vi "GetObjectivePosition.vi"(8 "error in (no error)":errorcluster) -> (0 "error out":errorcluster, 1 "output cluster":cluster{"X":dbl, "Y":dbl, "Z":dbl}, 2 "Valid":bool, 3 "CurrentPosition":cluster{"X":dbl, "Y":dbl, "Z":dbl, "Depth":dbl})   [LabVIEW 2014]
panel:
  out "Stale":bool
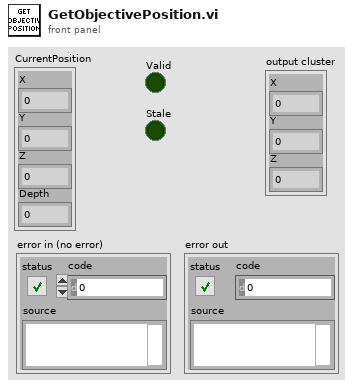
[diagram p1: front panel]
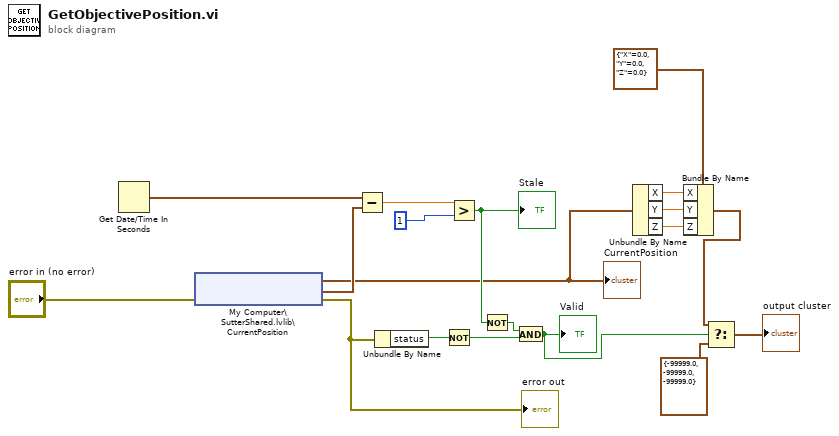
[diagram p0: block diagram]
diagram:
  n1 = Get Date/Time In Seconds() -> (seconds since 1Jan1904=w19:timestamp)
  n2 = shared-variable "My Computer\\SutterShared.lvlib\\CurrentPosition"(error in="error in (no error)") -> (w9:cluster{"X":dbl, "Y":dbl, "Z":dbl, "Depth":dbl}, error out=w13:errorcluster, w18:timestamp)
  "CurrentPosition" <- w9
  "error out" <- w13
  n3 = Subtract(x=w19, y=w18) -> (x-y=w17:dbl)
  n4 = Unbundle By Name(w13) -> ("status"=w11:bool)
  n5 = Not(x=w11) -> (.not. x?=w10:bool)
  n6 = Greater?(x=w17, y=1) -> (0:w14:bool)
  "Stale" <- w14
  n7 = Not(x=w14) -> (.not. x?=w12:bool)
  n8 = And(x=w12, y=w10) -> (x .and. y?=w4:bool)
  "Valid" <- w4
  n9 = Unbundle By Name(w9) -> ("X"=w8:dbl, "Y"=w7:dbl, "Z"=w6:dbl)
  n10 = Bundle By Name(cluster=cluster{"X":dbl, "Y":dbl, "Z":dbl} {"X"=0.0, "Y"=0.0, "Z"=0.0}, "X"=w8, "Y"=w7, "Z"=w6) -> (w3:cluster{"X":dbl, "Y":dbl, "Z":dbl})
  n11 = Select(t=w3, s=w4, f=cluster{"X":dbl, "Y":dbl, "Z":dbl} {"X"=-99999.0, "Y"=-99999.0, "Z"=-99999.0}) -> (s? t:f=→"output cluster":cluster{"X":dbl, "Y":dbl, "Z":dbl})
